vi "Potencia_+_Motor +OSA (1).vi"() -> ()   [LabVIEW 2014]
uses:
  <vilib>/DAQmx/read.llb/DAQmx Read (Analog DBL 1Chan 1Samp).vi
  <vilib>/DAQmx/create/channels.llb/DAQmx Create Channel (AI-Voltage-Basic).vi
  <vilib>/DAQmx/configure/timing.llb/DAQmx Timing (Sample Clock).vi
  <vilib>/Instr/_visa.llb/VISA Configure Serial Port (Instr).vi
  <vilib>/DAQmx/miscellaneous.llb/DAQmx Fill In Error Info.vi
  <vilib>/Utility/file.llb/Write To Spreadsheet File (DBL).vi
panel:
  out "Recibiendo información del OSA":bool
  out "Potencia":dbl[][](array[numeric])
  out "Distancia recorrida":dbl
  out "output array":dbl[][](array[numeric])
  in  "Distancia a recorrer (mm)":dbl=0.5
  in  "Ángulo":string(combo)
  in  "Stop":dbl=1570.0
  in  "Start":dbl=1470.0
  out "Respuesta OSA":string
  out "error out":errorcluster
  out "?":bool
  in  "Atributo":i32(listbox)
  in  "Blank/Disp":bool=TRUE
  in  "Sweep repeat":bool
  in  "Send":bool
  out "Espectro OSA":cluster{dbl[], dbl[]}(graph)
  in  "Trace":i32(listbox)
  in  "Preconfigurar":bool
  in  "Puerto":refnum<visa-resource-name>
  out "Potencia medida":dbl format="%0.2f"
  out "Gráfica de potencia":cluster{dbl[], dbl[]}(graph)
  in  "Índice de refracción":string="Potencia"
  out "size(s)":i32
  in  "Distancia inicial (mm)":dbl=124.65
  out "Tiempo X (S)":dbl
  out "Tiempo Y (S)":dbl format="%#_10g"
  out "Tiempo Z (S)":dbl
  in  "Start/Stop":bool
  in  "COM Config":T1={"VISA resource name"="COM4", "baud rate"=9600, "data bits"=8, "parity"=enum."None", "stop bits"=10, "flow control"=0} {"flow control" items=["None"=0, "XON/XOFF"=1, "RTS/CTS"=2, "DTR/DSR"=4]; "data bits" min=5 max=8 step=1}
  in  "COM Write":string="AA;\nVL0.0000,0.0100,0.0000;\nMR0.0000,-0.5000,0.0000;\nGO;"
  out "Waveform Chart":dbl(graph)
  in  "stop":bool
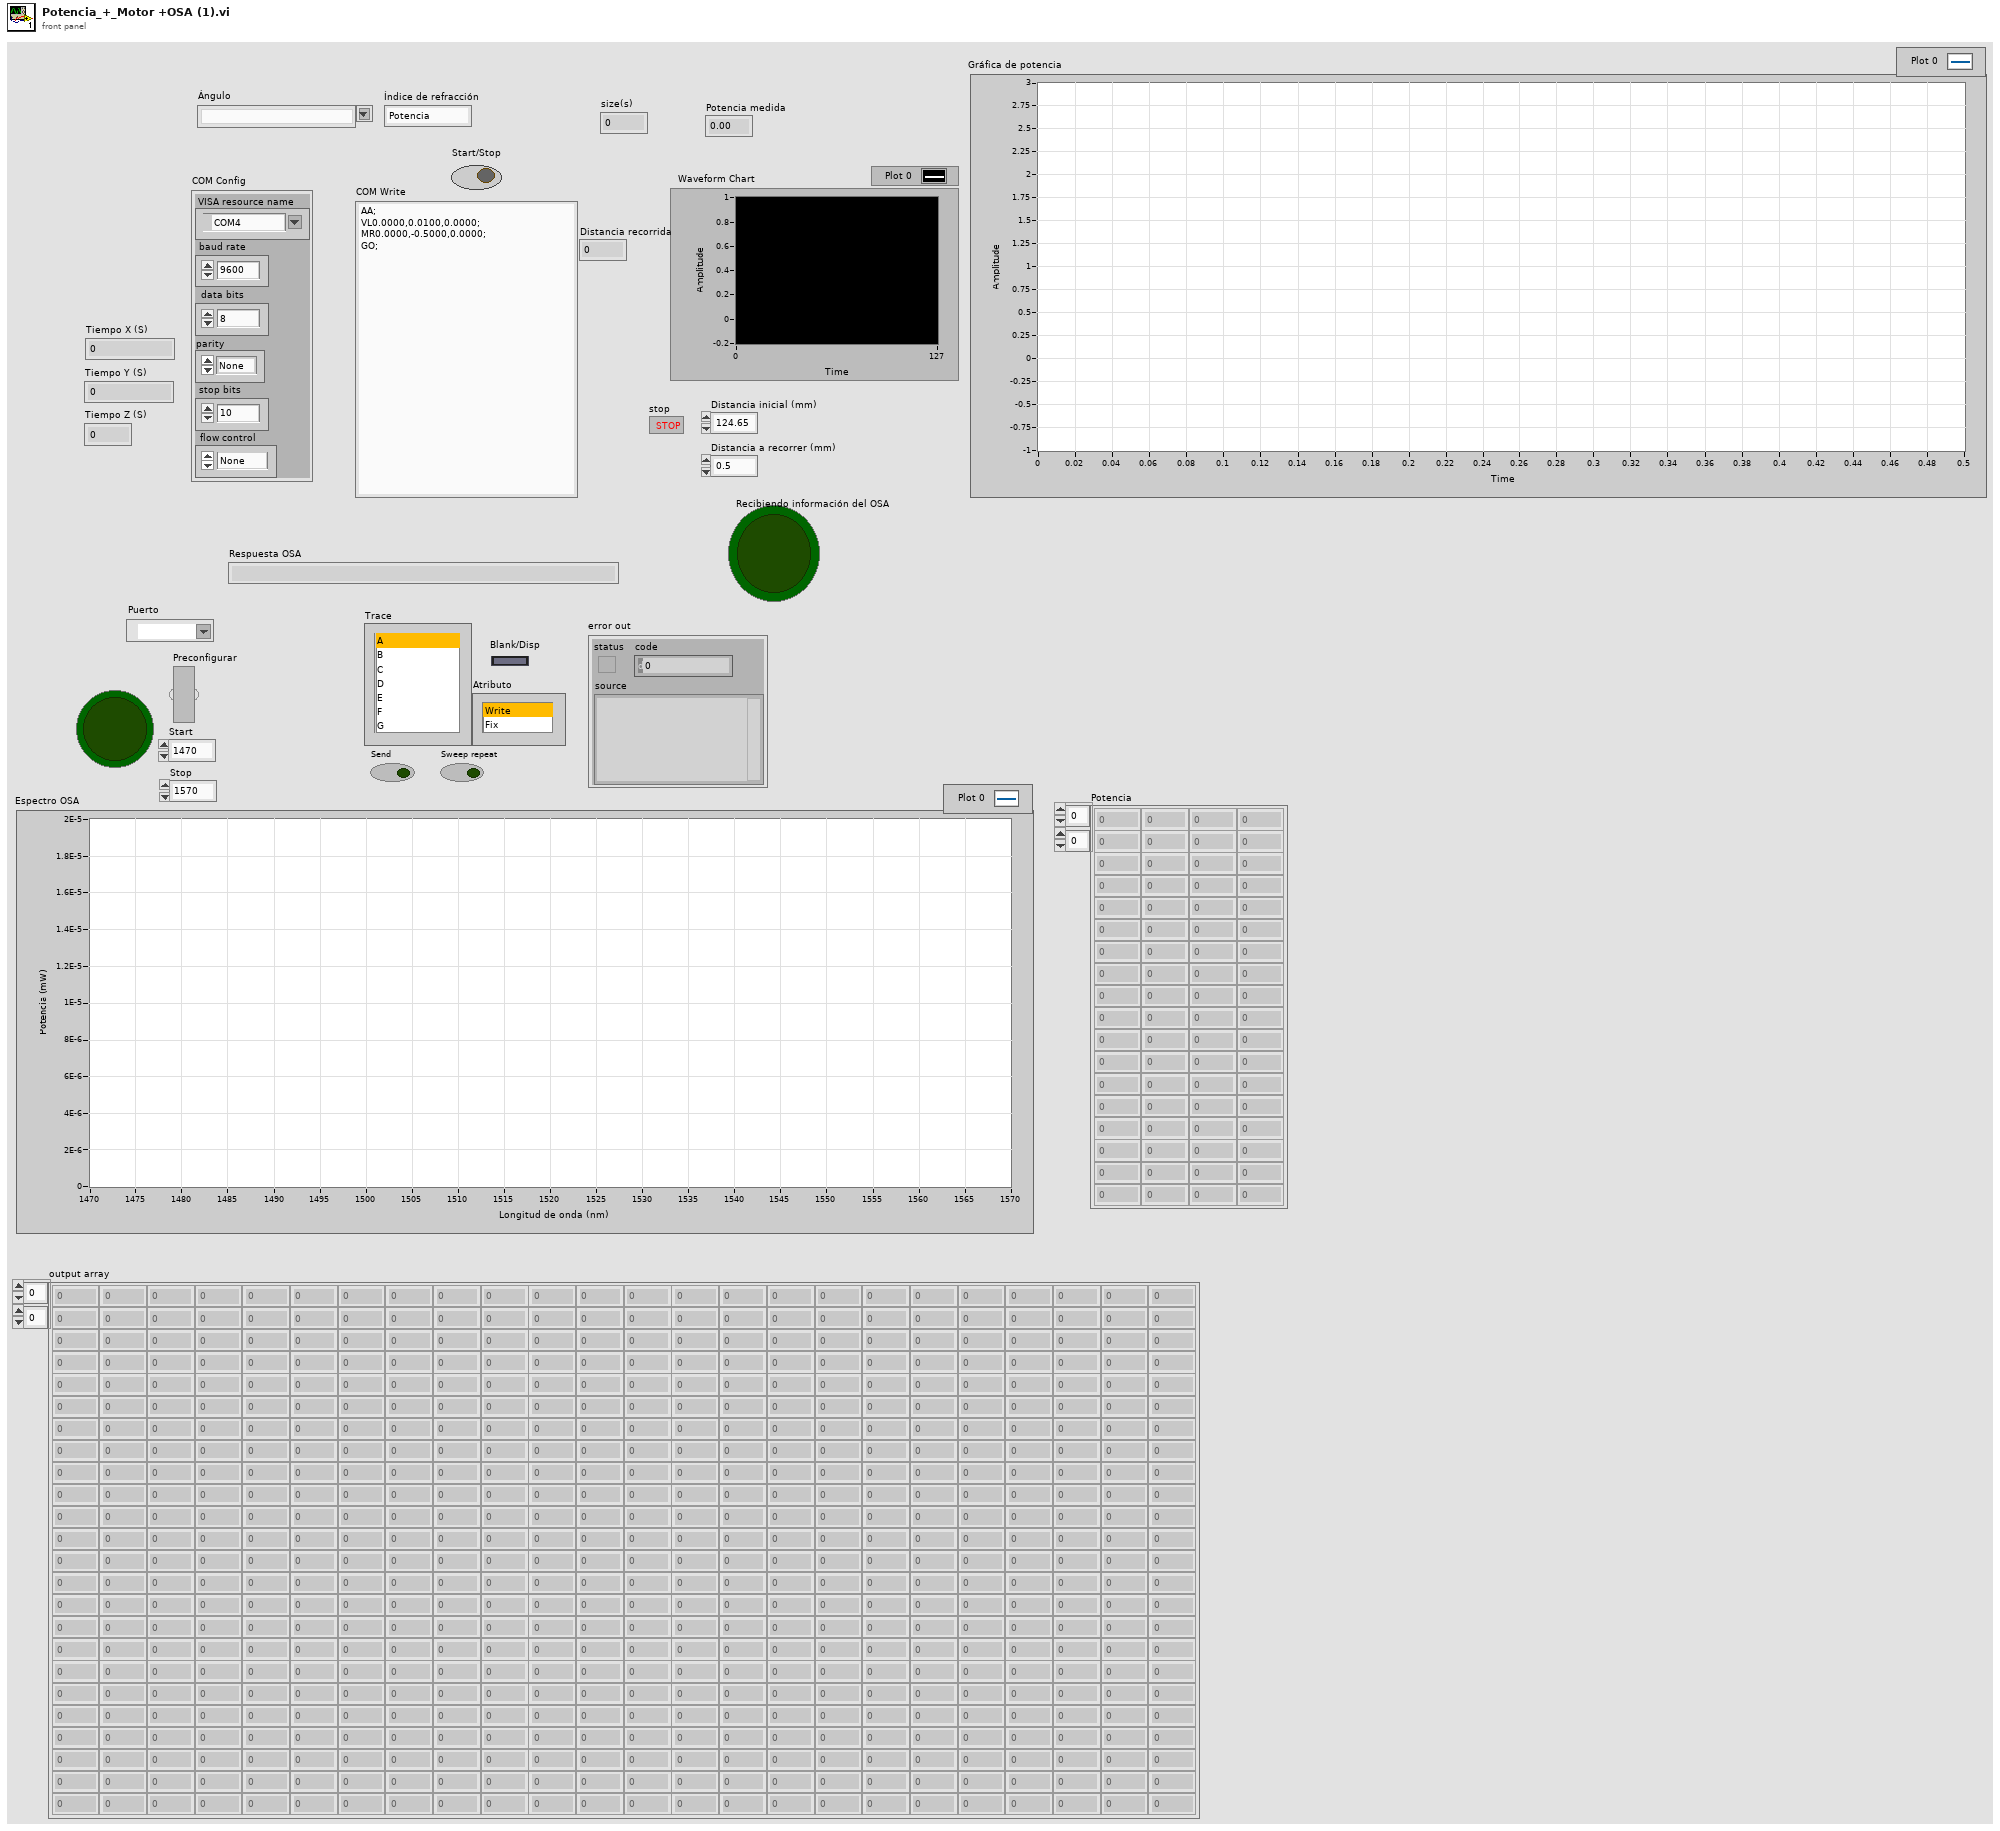
[diagram p1: front panel]
types:
  T1 = cluster{"VISA resource name":refnum<visa-resource-name>, "baud rate":u32, "data bits":u16, "parity":enum16{"None", "Odd", "Even", "Mark", "Space"}, "stop bits":u16, "flow control":u16}
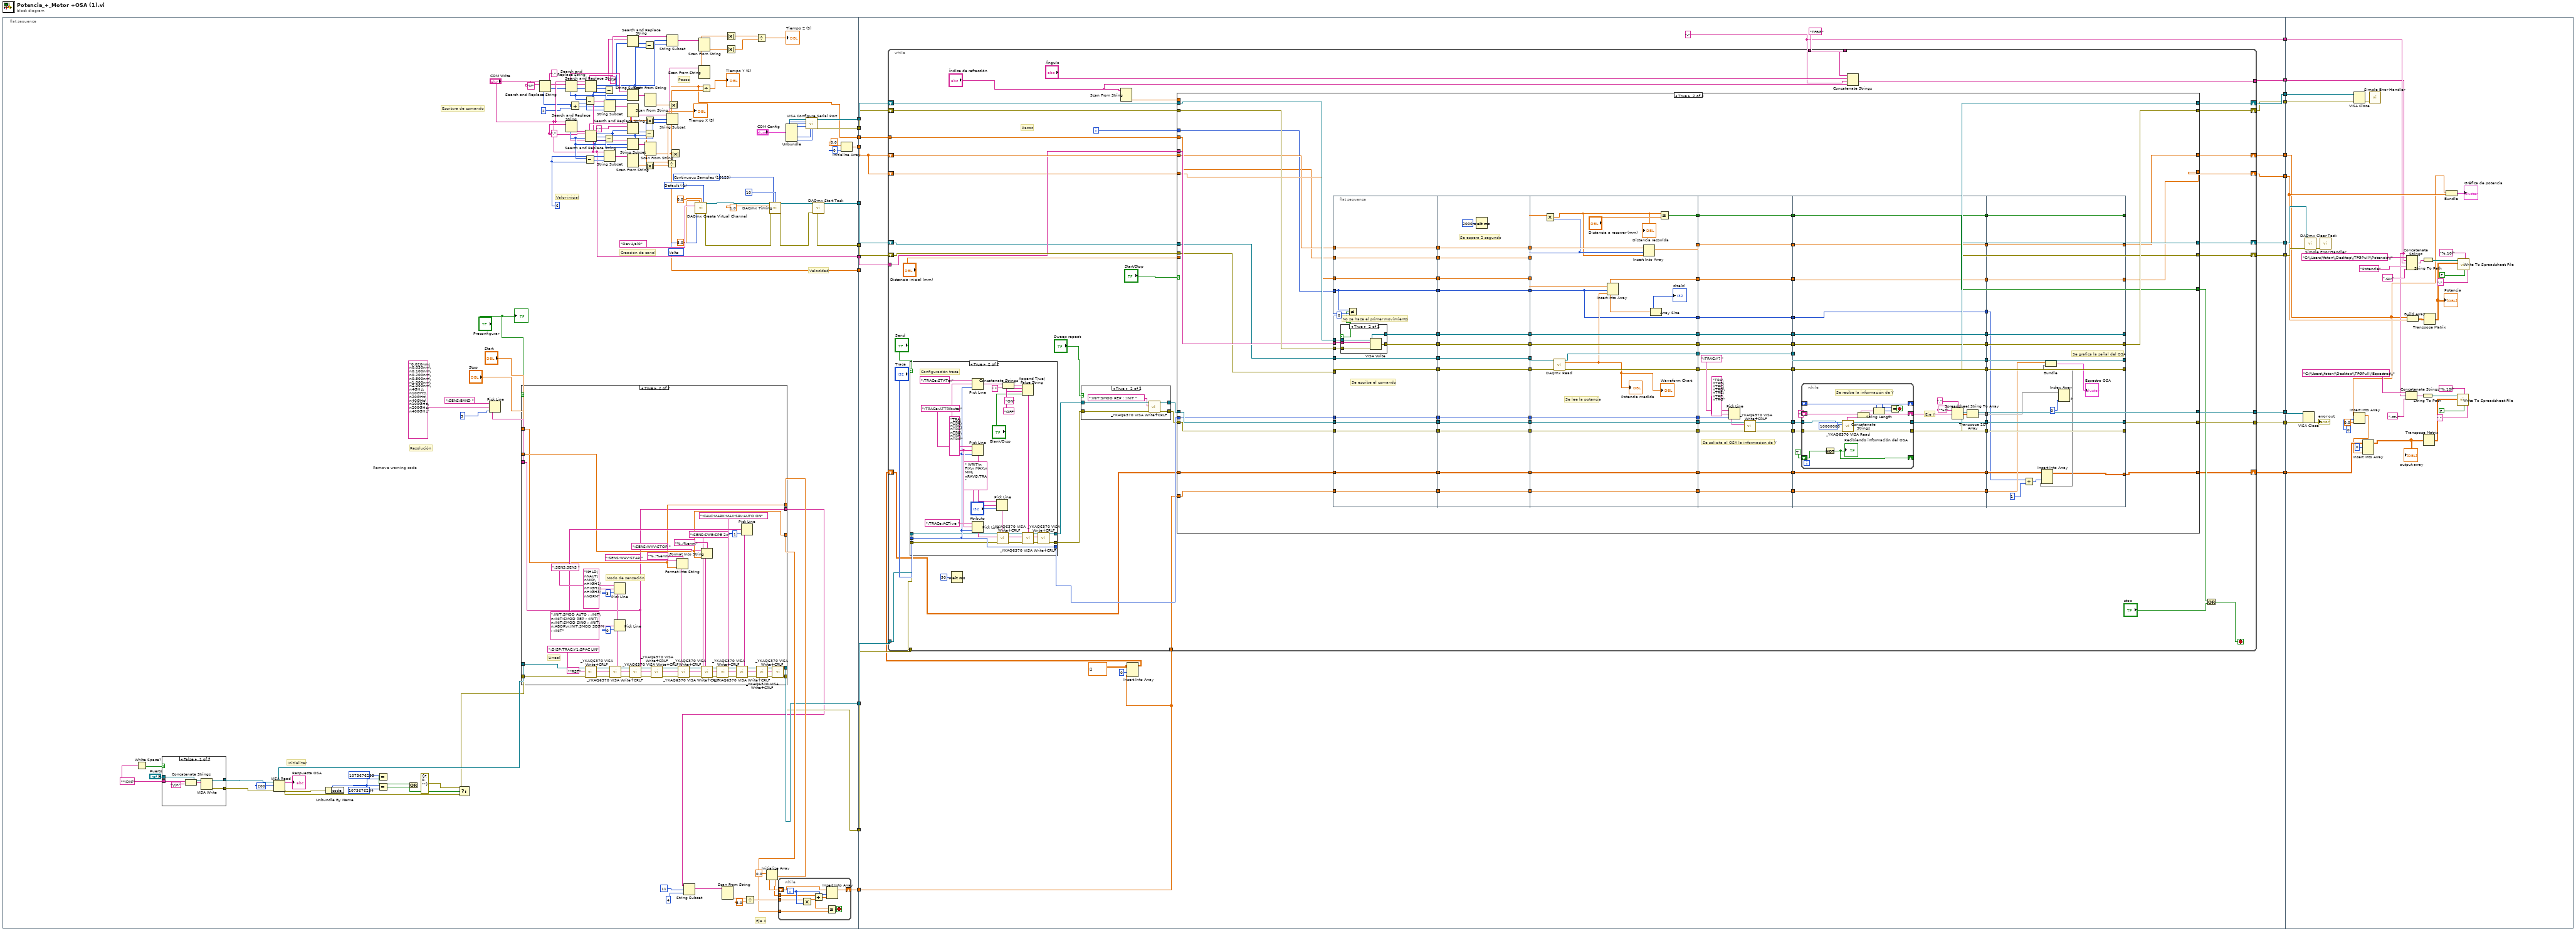
[diagram p0: block diagram]
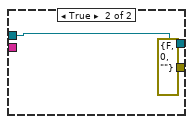
[diagram p3: hidden frame]
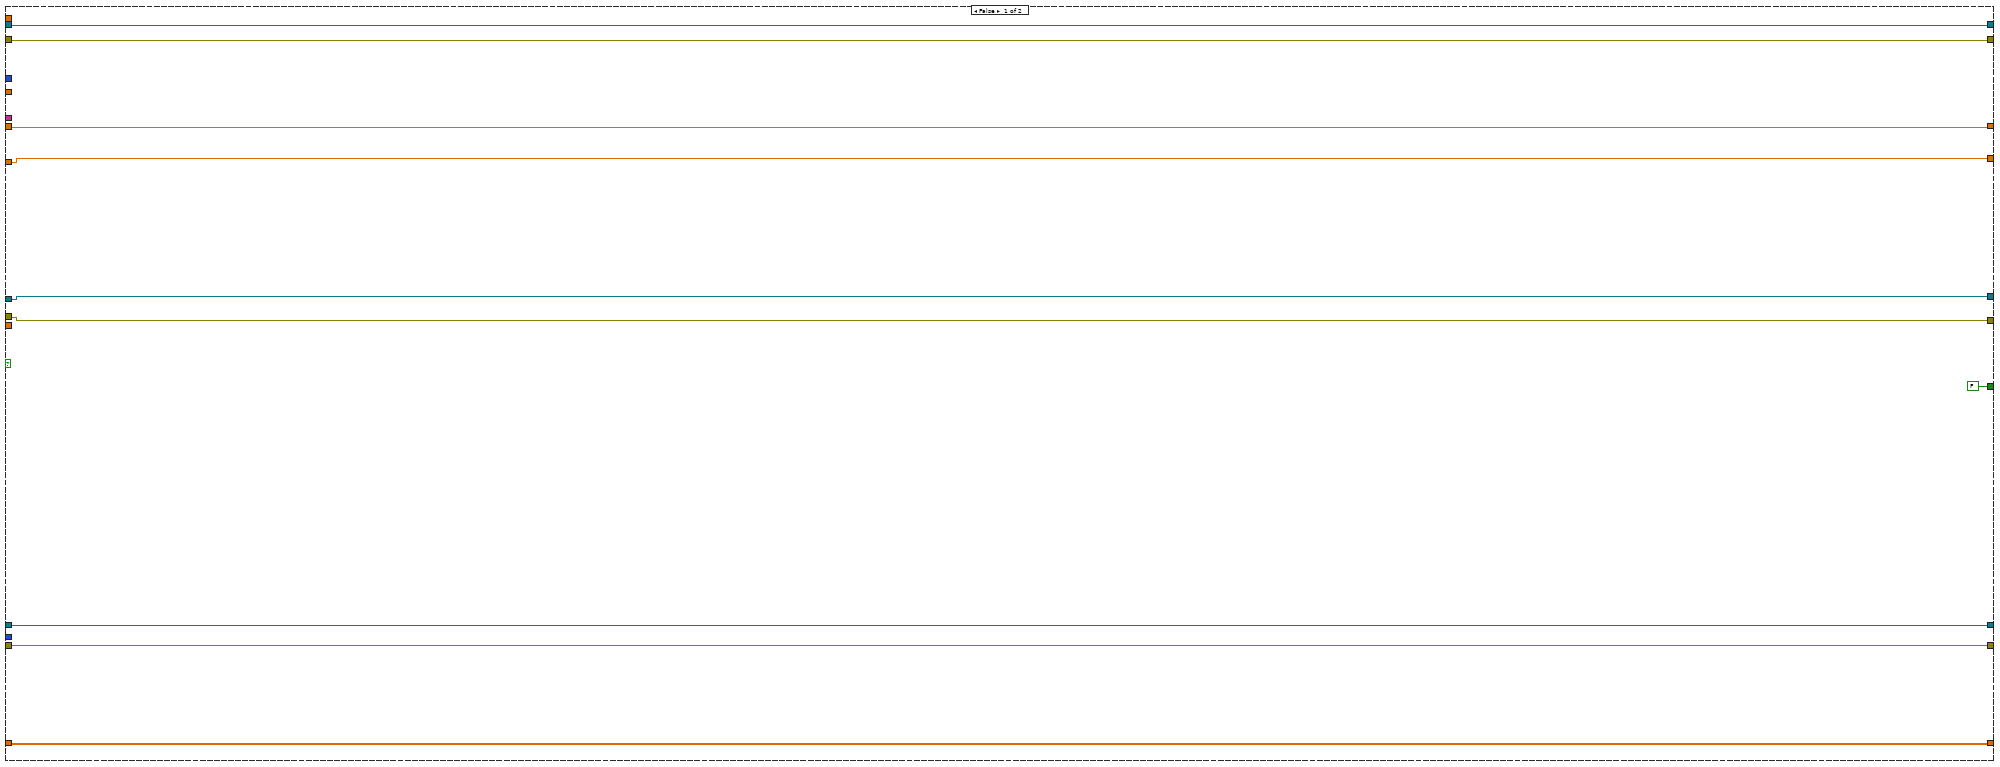
[diagram p6: hidden frame]
diagram:
  n1 = flat-sequence {
    tunnel: [w123] -> w22
    tunnel: [w122] -> w21
    tunnel: [w119] -> w20
    tunnel: [w111] -> w18
    tunnel: [w110] -> w17
    tunnel: ["COM Write"] -> w13
    tunnel: [w28] -> w10
    tunnel: [w27] -> w7
    tunnel: [w26] -> w6
    tunnel: [w25] -> w5
    tunnel: [w24] -> w3
    tunnel: w22 -> [w214]
    tunnel: w21 -> [w226]
    tunnel: w20 -> [w219]
    tunnel: [w218] -> w19
    tunnel: w18 -> [w225]
    tunnel: w17 -> [w224]
    tunnel: [w223] -> w16
    tunnel: [w222] -> w15
    tunnel: [w217] -> w14
    tunnel: w13 -> [w221]
    tunnel: [w216] -> w12
    tunnel: [w215] -> w11
    tunnel: w10 -> [_]
    tunnel: [w213] -> w9
    tunnel: [w212] -> w8
    tunnel: w7 -> [w206]
    tunnel: w6 -> [w211]
    tunnel: w5 -> [w210]
    tunnel: [w209] -> w4
    tunnel: w3 -> [w208]
    tunnel: [w203] -> w2
    tunnel: [w202] -> w1
    tunnel: w19 -> [w553]
    tunnel: w16 -> [w570]
    tunnel: w15 -> [w569]
    tunnel: w14 -> [w537]
    tunnel: w12 -> [w567]
    tunnel: w11 -> [w566]
    tunnel: w9 -> [w564]
    tunnel: w8 -> [w563]
    tunnel: w4 -> [w538]
    tunnel: w2 -> [w544]
    tunnel: w1 -> [w540]
    frame #0 {
      w50 = "*IDN?" ("Strings (empty)")
      w93 = "," ("search string")
      w103 = "," ("search string")
      w109 = 6 ("offset (0)")
      w126 = 10123 items=["Finite Samples"=10178, "Continuous Samples"=10123, "Hardware Timed Single Point"=12522] ("sample mode")
      w131 = -1 items=["Default"=-1, "RSE"=10083, "NRSE"=10078, "Differential"=10106, "Pseudodifferential"=12529] ("input terminal configuration")
      w134 = 10348 items=["Volts"=10348, "From Custom Scale"=10065] ("units")
      # "Pasos"
      # "Eje X"
      # "Resolución"
      # "Inizializar"
      # "Remove warning code"
      # "Velocidad"
      # "Escritura de comando"
      # "Valor inicial"
      # "Creación de canal"
      n2 = White Space?(1:w50) -> (0:w49:bool)
      n3 = case shown="False" w49 {
        tunnel: "Puerto" -> [w197 w201]
        tunnel: [w196 w201] -> w60
        tunnel: w50 -> [w195 _]
        tunnel: [w194 errorcluster {"status"=FALSE, "code"=0, "source"=""} ("error out")] -> w61
        frame False {
          n4 = Concatenate Strings(w195, "\r\n") -> (w198:string)
          n5 = VISA Write(VISA resource name=w197, write buffer=w198) -> (VISA resource name out=w196:refnum<visa-resource-name>, error out=w194:errorcluster)  [unwired: 1 in, 1 out]
        }
        frame True {
        }
      }
      n6 = VISA Read(VISA resource name=w60, byte count=u32 200 ("Byte Count (0)"), error in (no error)=w61) -> (VISA resource name out=w40:refnum<visa-resource-name>, read buffer=→"Respuesta OSA":string, error out=w53:errorcluster)  [unwired: 1 out]
      n7 = Unbundle By Name(w53) -> ("code"=w56:i32)
      n8 = Equal?(x=1073676293, y=w56) -> (x = y?=w57:bool)
      n9 = Equal?(x=1073676294, y=w56) -> (x = y?=w58:bool)
      n10 = Or(x=w57, y=w58) -> (x .or. y?=w59:bool)
      n11 = Select(t=errorcluster {"status"=FALSE, "code"=0, "source"=""}, s=w59, f=w53) -> (s? t:f=w39:errorcluster)
      n12 = Pick Line(string ("")=":SENS:BAND ", multi-line string="0.020nm\n0.050nm\n0.100nm\n0.200nm\n0.500nm\n1.000nm\n2.000nm\n4GHz\n10GHz\n20GHz\n40GHz\n100GHz\n200GHz\n400GHz", line index=3) -> (output string=w47:string)
      n13 = case shown="True" "Preconfigurar" {
        tunnel: w40 -> [w149 w192]
        tunnel: w39 -> [w148 w191]
        tunnel: [w149 w157] -> w26
        tunnel: [w148 w156] -> w25
        tunnel: [w145 w150] -> w23
        tunnel: [w147 w151] -> w30
        tunnel: [w146 w152] -> w29
        tunnel: "Stop" -> [w146 w152]
        tunnel: "Start" -> [w147 w151]
        tunnel: w47 -> [w145 w150]
        frame False {
        }
        frame True {
          w168 = ":INIT:SMOD AUTO ; :INIT\n:INIT:SMOD REP ; :INIT\n:INIT:SMOD SING ; :INIT\n:ABOR\n:INIT:SMOD SEGM ; :INIT"
          # "Lineal"
          # "Modo de sensación"
          n14 = call <instrlib>:"_YKAQ6370 VISA Write+CRLF.vi"("error in (no error)"=w191, "Strings (empty)"="*RST", "VISA resource name"=w192) -> ("error out"=w163:errorcluster, "VISA resource name out"=w164:refnum<visa-resource-name>)  [unwired: 7 in]
          n15 = call <instrlib>:"_YKAQ6370 VISA Write+CRLF.vi"("error in (no error)"=w163, "Strings (empty)"=":DISP:TRAC:Y1:SPAC LIN", "VISA resource name"=w164) -> ("error out"=w160:errorcluster, "VISA resource name out"=w161:refnum<visa-resource-name>)  [unwired: 7 in]
          n16 = Pick Line(string ("")=":SENS:SENS ", multi-line string="NHLD\nNAUT\nMID\nHIGH1\nHIGH2\nHIGH3\nNORM", line index=3) -> (output string=w184:string)
          n17 = Pick Line(multi-line string=w168, line index=0) -> (output string=w172:string)  [unwired: 1 in]
          n18 = call <instrlib>:"_YKAQ6370 VISA Write+CRLF.vi"("error in (no error)"=w160, "Strings (empty)"=w172, "VISA resource name"=w161) -> ("error out"=w173:errorcluster, "VISA resource name out"=w174:refnum<visa-resource-name>)  [unwired: 7 in]
          n19 = call <instrlib>:"_YKAQ6370 VISA Write+CRLF.vi"("error in (no error)"=w173, "Strings (empty)"=w150, "VISA resource name"=w174) -> ("error out"=w188:errorcluster, "VISA resource name out"=w187:refnum<visa-resource-name>)  [unwired: 7 in]
          n20 = Format Into String(format string="%.;%enm", initial string=":SENS:WAV:STAR ", w151) -> (resulting string=w178:string)  [unwired: 1 in, 1 out]
          n21 = call <instrlib>:"_YKAQ6370 VISA Write+CRLF.vi"("error in (no error)"=w188, "Strings (empty)"=w184, "VISA resource name"=w187) -> ("error out"=w189:errorcluster, "VISA resource name out"=w190:refnum<visa-resource-name>)  [unwired: 7 in]
          n22 = Format Into String(format string="%.;%enm", initial string=":SENS:WAV:STOP ", w152) -> (resulting string=w176:string)  [unwired: 1 in, 1 out]
          n23 = call <instrlib>:"_YKAQ6370 VISA Write+CRLF.vi"("error in (no error)"=w189, "Strings (empty)"=w178, "VISA resource name"=w190) -> ("error out"=w181:errorcluster, "VISA resource name out"=w182:refnum<visa-resource-name>)  [unwired: 7 in]
          n24 = call <instrlib>:"_YKAQ6370 VISA Write+CRLF.vi"("error in (no error)"=w181, "Strings (empty)"=w176, "VISA resource name"=w182) -> ("error out"=w158:errorcluster, "VISA resource name out"=w159:refnum<visa-resource-name>)  [unwired: 7 in]
          n25 = call <instrlib>:"_YKAQ6370 VISA Write+CRLF.vi"("error in (no error)"=w158, "Strings (empty)"=":SENS:SWE:SPE 2x", "VISA resource name"=w159) -> ("error out"=w166:errorcluster, "VISA resource name out"=w167:refnum<visa-resource-name>)  [unwired: 7 in]
          n26 = Pick Line(multi-line string=w168, line index=1) -> (output string=w169:string)  [unwired: 1 in]
          n27 = call <instrlib>:"_YKAQ6370 VISA Write+CRLF.vi"("error in (no error)"=w166, "Strings (empty)"=w169, "VISA resource name"=w167) -> ("error out"=w154:errorcluster, "VISA resource name out"=w155:refnum<visa-resource-name>)  [unwired: 7 in]
          n28 = call <instrlib>:"_YKAQ6370 VISA Write+CRLF.vi"("error in (no error)"=w154, "Strings (empty)"=":CALC:MARK:MAX:SRL:AUTO ON", "VISA resource name"=w155) -> ("error out"=w156:errorcluster, "VISA resource name out"=w157:refnum<visa-resource-name>)  [unwired: 7 in]
        }
      }
      n29 = Search and Replace String(input string="COM Write", search string="M" ("replace string (\"\")")) -> (offset past replacement=w84:i32)  [unwired: 6 in, 3 out]
      n30 = Search and Replace String(input string="COM Write", search string=w93, offset=w84) -> (result string=w95:string, offset past replacement=w96:i32)  [unwired: 5 in, 2 out]
      n31 = Search and Replace String(input string="COM Write", search string=w103) -> (result string=w105:string, offset past replacement=w106:i32)  [unwired: 6 in, 2 out]
      n32 = Add(x=w84, y=2) -> (x+y=w82:i32)
      n33 = Subtract(x=w96, y=w82) -> (x-y=w85:i32)
      n34 = Subtract(x=w106, y=w109) -> (x-y=w108:i32)
      n35 = Search and Replace String(input string=w95, search string=w93, offset=w96) -> (result string=w94:string, offset past replacement=w89:i32)  [unwired: 5 in, 2 out]
      n36 = Search and Replace String(input string=w105, search string=w103, offset=w106) -> (result string=w104:string, offset past replacement=w99:i32)  [unwired: 5 in, 2 out]
      n37 = Subtract(x=w89, y=w96) -> (x-y=w97:i32)
      n38 = Subtract(x=w99, y=w106) -> (x-y=w107:i32)
      n39 = String Subset(string="COM Write", offset (0)=w82, length (rest)=w85) -> (substring=w64:string)
      n40 = String Subset(string="COM Write", offset (0)=w109, length (rest)=w108) -> (substring=w63:string)
      n41 = Search and Replace String(input string=w94, search string=";", offset=w89) -> (result string=w92:string, offset past replacement=w90:i32)  [unwired: 5 in, 2 out]
      n42 = String Subset(string=w95, offset (0)=w96, length (rest)=w97) -> (substring=w68:string)
      n43 = Scan From String(input string=w64) -> (output 1=w76:dbl)  [unwired: 4 in, 3 out]
      n44 = Search and Replace String(input string=w104, search string=";", offset=w99) -> (result string=w102:string, offset past replacement=w100:i32)  [unwired: 5 in, 2 out]
      n45 = String Subset(string=w105, offset (0)=w106, length (rest)=w107) -> (substring=w67:string)
      n46 = Scan From String(input string=w63) -> (output 1=w79:dbl)  [unwired: 4 in, 3 out]
      n47 = Subtract(x=w90, y=w89) -> (x-y=w91:i32)
      n48 = Subtract(x=w100, y=w99) -> (x-y=w101:i32)
      n49 = Absolute Value(x=w76) -> (abs(x)=w77:dbl)
      n50 = Absolute Value(x=w79) -> (abs(x)=w78:dbl)
      n51 = Scan From String(input string=w68) -> (output 1=w71:dbl)  [unwired: 4 in, 3 out]
      n52 = Scan From String(input string=w67) -> (output 1=w70:dbl)  [unwired: 4 in, 3 out]
      n53 = Divide(x=w77, y=w78) -> (x/y=→"Tiempo X (S)":dbl)
      n54 = String Subset(string=w92, offset (0)=w89, length (rest)=w91) -> (substring=w66:string)
      n55 = String Subset(string=w102, offset (0)=w99, length (rest)=w101) -> (substring=w65:string)
      n56 = Absolute Value(x=w71) -> (abs(x)=w24:dbl)
      n57 = Absolute Value(x=w70) -> (abs(x)=w28:dbl)
      n58 = String Subset(string=w23, offset (0)=11, length (rest)=4 ("length (rest)")) -> (substring=w37:string)
      n59 = call-poly <vilib>:"DAQmx Create Virtual Channel.vi"("maximum value"=5.0, "minimum value"=0.0, "input terminal configuration"=w131, "physical channels"=tag "Dev4/ai0", "units"=w134) -> ("task out"=w130:refnum<k21>, "error out"=w129:errorcluster)  [unwired: 9 in]
      n60 = Scan From String(input string=w66) -> (output 1=w75:dbl)  [unwired: 4 in, 3 out]
      n61 = Scan From String(input string=w65) -> (output 1=w73:dbl)  [unwired: 4 in, 3 out]
      n62 = Divide(x=w24, y=w28) -> (x/y=→"Tiempo Y (S)":dbl)
      n63 = Scan From String(input string=w37) -> (output 1=w33:dbl)  [unwired: 4 in, 3 out]
      n64 = Absolute Value(x=w75) -> (abs(x)=w74:dbl)
      n65 = Absolute Value(x=w73) -> (abs(x)=w72:dbl)
      n66 = Divide(x=w33, y=5.0) -> (x/y=w32:dbl)
      n67 = Divide(x=w74, y=w72) -> (x/y=→"Tiempo Z (S)":dbl)
      n68 = Initialize Array(0.0 ("element")) -> (w36:dbl[])  [unwired: 1 in]
      n69 = call-poly <vilib>:"DAQmx Timing.vi"("task/channels in"=w130, "sample mode"=w126, "samples per channel"=10, "rate"=1.0, "error in"=w129) -> ("task out"=w125:refnum<k21>, "error out"=w124:errorcluster)  [unwired: 9 in]
      n70 = while {
        shift-right: [w143] -> w27
        shift-left: w36 -> [w144]
        tunnel: w30 -> [w139]
        tunnel: w32 -> [w141]
        tunnel: w29 -> [w137]
        i -> [w142]
        stop <- w136 stop-if-true
        n71 = Multiply(x=w141, y=w142) -> (x*y=w140:dbl)
        n72 = Add(x=w139, y=w140) -> (x+y=w138:dbl)
        n73 = Greater Or Equal?(x=w138, y=w137) -> (x >= y?=w136:bool)
        n74 = Insert Into Array(array=w144, index=w142, new element=w138) -> (w143:dbl[])
      }
      n75 = Unbundle("COM Config") -> ("VISA resource name"=w113:refnum<visa-resource-name>, "baud rate"=w114:u32, "data bits"=w115:u16, "parity"=w118:enum16{"None", "Odd", "Even", "Mark", "Space"}, "stop bits"=w116:u16, "flow control"=w117:u16)
      n76 = call-poly "VISA Configure Serial Port"("VISA resource name"=w113, "baud rate (9600)"=w114, "data bits (8)"=w115, "parity (0:none)"=w118, "stop bits (10: 1 bit)"=w116, "flow control (0:none)"=w117) -> ("VISA resource name out"=w111:refnum<visa-resource-name>, "error out"=w110:errorcluster)  [unwired: 8 in]
      n77 = call <vilib>:"DAQmx Start Task.vi"("task/channels in"=w125, "error in"=w124) -> ("task out"=w123:refnum<k21>, "error out"=w122:errorcluster)  [unwired: 12 in]
      n78 = Initialize Array(0.0 ("element"), 0 ("dimension size")) -> (w119:dbl[])
      "?" <- "Preconfigurar"
    }
    frame #1 {
      w202 = "-"
      n79 = Insert Into Array(array=dbl[][] [], index (col)=0 ("disabled index (col)"), new element=w206) -> (w204:dbl[][])  [unwired: 1 in]
      n80 = while {
        shift-right: [w253] -> w217
        shift-left: w219 -> [w268]
        shift-right: [w265] -> w223
        shift-left: w225 -> [w262]
        shift-right: [w264] -> w222
        shift-left: w224 -> [w266]
        tunnel: w221 -> [w261]
        tunnel: [w256] -> w209
        tunnel: "TFBG" -> [w259]
        tunnel: w202 -> [w257]
        shift-right: [w254] -> w218
        shift-left: w219 -> [w255]
        shift-right: [w252] -> w216
        shift-left: w214 -> [w250]
        shift-right: [w251] -> w215
        shift-left: w226 -> [w267]
        tunnel: [w242] -> w213
        tunnel: [w241] -> w212
        tunnel: w211 -> [w240]
        tunnel: w210 -> [w239]
        tunnel: w208 -> [w237]
        tunnel: w206 -> [w231]
        shift-right: [w230] -> w203
        shift-left: w204 -> [w229]
        i -> [w236]
        stop <- w233 stop-if-true
        # "Pasos"
        n81 = case shown="True" "Send" {
          tunnel: [w277 w284] -> w238
          tunnel: [w276 w283] -> w248
          tunnel: [w278 w281] -> w243
          tunnel: "Trace" -> [w278 w281]
          tunnel: w240 -> [w277 w280]
          tunnel: w239 -> [w276 w279]
          frame False {
          }
          frame True {
            w286 = "TRA\nTRB\nTRC\nTRD\nTRE\nTRF\nTRG"
            # "Configuración trace"
            n82 = Pick Line(string ("")=":TRACe:STATe:", multi-line string=w286, line index=w281) -> (output string=w287:string)
            n83 = Pick Line(string ("")=":TRACe:ATTRibute:", multi-line string=w286, line index=w281) -> (output string=w292:string)
            n84 = Pick Line(string ("")=":TRACe:ACTive ", multi-line string=w286, line index=w281) -> (output string=w288:string)
            n85 = Pick Line(string ("")=w292, multi-line string=" WRIT\n FIX\n MAX\n MIN\nRAVG:TRA ", line index="Atributo") -> (output string=w291:string)
            n86 = call <instrlib>:"_YKAQ6370 VISA Write+CRLF.vi"("error in (no error)"=w279, "Strings (empty)"=w288, "VISA resource name"=w280) -> ("error out"=w300:errorcluster, "VISA resource name out"=w299:refnum<visa-resource-name>)  [unwired: 7 in]
            n87 = Concatenate Strings(w287, " " ("string")) -> (w290:string)
            n88 = Append True/False String(1:"Blank/Disp", 2:"OFF", 3:"ON", 4:w290) -> (0:w296:string)
            n89 = call <instrlib>:"_YKAQ6370 VISA Write+CRLF.vi"("error in (no error)"=w300, "Strings (empty)"=w291, "VISA resource name"=w299) -> ("error out"=w297:errorcluster, "VISA resource name out"=w298:refnum<visa-resource-name>)  [unwired: 7 in]
            n90 = call <instrlib>:"_YKAQ6370 VISA Write+CRLF.vi"("error in (no error)"=w297, "Strings (empty)"=w296, "VISA resource name"=w298) -> ("error out"=w283:errorcluster, "VISA resource name out"=w284:refnum<visa-resource-name>)  [unwired: 7 in]
          }
        }
        n91 = Wait (ms)(milliseconds to wait=u32 50) -> ()  [unwired: 1 out]
        n92 = case shown="True" "Sweep repeat" {
          tunnel: w238 -> [w270 w275]
          tunnel: w248 -> [w269 w274]
          tunnel: [w270 w272] -> w244
          tunnel: [w269 w271] -> w232
          frame False {
          }
          frame True {
            n93 = call <instrlib>:"_YKAQ6370 VISA Write+CRLF.vi"("error in (no error)"=w274, "Strings (empty)"=":INIT:SMOD REP ; :INIT ", "VISA resource name"=w275) -> ("error out"=w271:errorcluster, "VISA resource name out"=w272:refnum<visa-resource-name>)  [unwired: 7 in]
          }
        }
        n94 = Scan From String(input string="Índice de refracción") -> (output 1=w228:dbl)  [unwired: 4 in, 3 out]
        n95 = case shown="True" "Start/Stop" {
          tunnel: w250 -> [w311 w382]
          tunnel: w268 -> [w308 w367]
          tunnel: w267 -> [w310 w381]
          tunnel: [w309 w371] -> w254
          tunnel: w262 -> [w313 w391]
          tunnel: w266 -> [w312 w390]
          tunnel: [w313 w384] -> w265
          tunnel: [w312 w383] -> w264
          tunnel: [w308 w368] -> w253
          tunnel: w261 -> [_ w389]
          tunnel: "Distancia inicial (mm)" -> [_ _]
          tunnel: w255 -> [w309 w374]
          tunnel: [w311 w376] -> w252
          tunnel: [w310 w375] -> w251
          tunnel: w244 -> [w307 w399]
          tunnel: w232 -> [w306 w398]
          tunnel: w243 -> [_ w397]
          tunnel: [w307 w396] -> w242
          tunnel: [w306 w395] -> w241
          tunnel: w237 -> [_ w365]
          tunnel: w236 -> [_ w366]
          tunnel: [FALSE w362] -> w234
          tunnel: w229 -> [w304 w329]
          tunnel: w231 -> [_ w328]
          tunnel: [w304 w314] -> w230
          tunnel: w228 -> [_ _]
          frame False {
          }
          frame True {
            n96 = flat-sequence {
              tunnel: w397 -> [w417]
              tunnel: w398 -> [w418]
              tunnel: w399 -> [w419]
              tunnel: [w419] -> w361
              tunnel: [w418] -> w359
              tunnel: [w417] -> w357
              tunnel: w391 -> [w416]
              tunnel: w390 -> [w415]
              tunnel: w389 -> [w414]
              tunnel: [w413] -> w355
              tunnel: [w412] -> w353
              tunnel: w382 -> [w411]
              tunnel: [w411] -> w351
              tunnel: w381 -> [w410]
              tunnel: [w410] -> w349
              tunnel: w374 -> [w409]
              tunnel: [w409] -> w347
              tunnel: w367 -> [w408]
              tunnel: [w408] -> w345
              tunnel: w366 -> [w406]
              tunnel: [w406] -> w343
              tunnel: w365 -> [w407]
              tunnel: [w407] -> w341
              tunnel: w329 -> [w402]
              tunnel: w328 -> [w403]
              tunnel: [w403] -> w323
              tunnel: [w402] -> w318
              tunnel: w361 -> [w440]
              tunnel: [w440] -> w360
              tunnel: w359 -> [w439]
              tunnel: [w439] -> w358
              tunnel: w357 -> [w438]
              tunnel: [w438] -> w356
              tunnel: w355 -> [w437]
              tunnel: [w437] -> w354
              tunnel: w353 -> [w436]
              tunnel: [w436] -> w352
              tunnel: w351 -> [w435]
              tunnel: [w435] -> w350
              tunnel: w349 -> [w434]
              tunnel: [w434] -> w348
              tunnel: w347 -> [w433]
              tunnel: [w433] -> w346
              tunnel: w345 -> [w432]
              tunnel: [w432] -> w344
              tunnel: w343 -> [w431]
              tunnel: [w431] -> w342
              tunnel: w341 -> [w430]
              tunnel: [w430] -> w340
              tunnel: [w428] -> w324
              tunnel: w323 -> [w428]
              tunnel: [w427] -> w319
              tunnel: w318 -> [w427]
              tunnel: [w462] -> w394
              tunnel: [w461] -> w393
              tunnel: [w460] -> w392
              tunnel: w360 -> [w462]
              tunnel: w358 -> [w461]
              tunnel: w356 -> [w460]
              tunnel: [w459] -> w387
              tunnel: w354 -> [w459]
              tunnel: [w458] -> w385
              tunnel: w352 -> [w458]
              tunnel: w350 -> [w457]
              tunnel: w348 -> [w456]
              tunnel: [w455] -> w379
              tunnel: [w454] -> w377
              tunnel: w346 -> [w453]
              tunnel: [w451] -> w372
              tunnel: w344 -> [w449]
              tunnel: [w448] -> w369
              tunnel: w342 -> [w442]
              tunnel: w340 -> [w446]
              tunnel: [w445] -> w363
              tunnel: [w444] -> w325
              tunnel: w324 -> [w444]
              tunnel: [w443] -> w320
              tunnel: w319 -> [w443]
              tunnel: [w442] -> w315
              tunnel: [w478] -> w401
              tunnel: [w477] -> w400
              tunnel: w394 -> [w480]
              tunnel: w393 -> [w479]
              tunnel: w392 -> [w473]
              tunnel: [w472] -> w388
              tunnel: w387 -> [w472]
              tunnel: [w471] -> w386
              tunnel: w385 -> [w471]
              tunnel: [w470] -> w380
              tunnel: w379 -> [w470]
              tunnel: [w469] -> w378
              tunnel: w377 -> [w469]
              tunnel: [w468] -> w373
              tunnel: w372 -> [w468]
              tunnel: [w467] -> w370
              tunnel: w369 -> [w467]
              tunnel: [w466] -> w364
              tunnel: w363 -> [w466]
              tunnel: [w465] -> w326
              tunnel: w325 -> [w465]
              tunnel: [w464] -> w321
              tunnel: w320 -> [w464]
              tunnel: [w463] -> w316
              tunnel: w315 -> [w463]
              tunnel: w401 -> [w501]
              tunnel: w400 -> [w500]
              tunnel: w388 -> [w491]
              tunnel: w386 -> [w490]
              tunnel: w380 -> [w489]
              tunnel: w378 -> [w488]
              tunnel: w373 -> [w487]
              tunnel: w370 -> [w486]
              tunnel: w364 -> [w485]
              tunnel: [w494] -> w339
              tunnel: [w493] -> w338
              tunnel: [w492] -> w337
              tunnel: [w491] -> w336
              tunnel: [w490] -> w335
              tunnel: [w489] -> w334
              tunnel: [w488] -> w333
              tunnel: [w487] -> w332
              tunnel: [w486] -> w331
              tunnel: [w485] -> w330
              tunnel: [w484] -> w327
              tunnel: w326 -> [w484]
              tunnel: [w483] -> w322
              tunnel: w321 -> [w483]
              tunnel: [w482] -> w317
              tunnel: w316 -> [w482]
              tunnel: [w525] -> w362
              tunnel: [w526] -> w368
              tunnel: [w527] -> w371
              tunnel: [w528] -> w375
              tunnel: [w529] -> w376
              tunnel: [w530] -> w383
              tunnel: [w531] -> w384
              tunnel: [w532] -> w395
              tunnel: [w533] -> w396
              tunnel: w339 -> [w524]
              tunnel: w338 -> [w533]
              tunnel: w337 -> [w532]
              tunnel: w336 -> [w531]
              tunnel: w335 -> [w530]
              tunnel: w334 -> [w529]
              tunnel: w333 -> [w528]
              tunnel: w332 -> [w527]
              tunnel: w331 -> [w526]
              tunnel: w330 -> [w525]
              tunnel: w327 -> [w522]
              tunnel: w322 -> [w520]
              tunnel: w317 -> [w518]
              tunnel: [w516] -> w314
              frame #0 {
                # "No se hace el primer movimiento"
                # "Se escribe el comando"
                n97 = Not Equal?(x=w406, y=0) -> (x != y?=w404:bool)
                n98 = case shown="True" w404 {
                  tunnel: w416 -> [w421 w426]
                  tunnel: w415 -> [w420 w425]
                  tunnel: w414 -> [_ w424]
                  tunnel: [w421 w423] -> w413
                  tunnel: [w420 w422] -> w412
                  frame False {
                  }
                  frame True {
                    n99 = VISA Write(VISA resource name=w426, write buffer=w424, error in (no error)=w425) -> (VISA resource name out=w423:refnum<visa-resource-name>, error out=w422:errorcluster)  [unwired: 1 out]
                  }
                }
              }
              frame #1 {
                # "Se espera 2 segundo"
                n100 = Wait (ms)(milliseconds to wait=u32 2000) -> ()  [unwired: 1 out]
              }
              frame #2 {
                # "Se lee la potencia"
                n101 = Multiply(x=w446, y=w442) -> (x*y=w441:dbl)
                "Distancia recorrida" <- w441
                n102 = call-poly <vilib>:"DAQmx Read.vi"("task/channels in"=w457, "error in"=w456) -> ("task out"=w455:refnum<k21>, "data"=w450:dbl, "error out"=w454:errorcluster)  [unwired: 11 in]
                "Potencia medida" <- w450
                "Waveform Chart" <- w450
                n103 = Insert Into Array(array=w453, index=w442, new element=w450) -> (w451:dbl[])
                n104 = Insert Into Array(array=w449, index=w442, new element=w441) -> (w448:dbl[])
                n105 = Array Size(array=w451) -> (size(s)=→"size(s)":i32)
                n106 = Greater Or Equal?(x=w441, y="Distancia a recorrer (mm)") -> (x >= y?=w445:bool)
              }
              frame #3 {
                # "Se solicita al OSA la información de Y"
                n107 = Pick Line(string ("")=":TRAC:Y? " ("Strings (empty)"), multi-line string="TRA\nTRB\nTRC\nTRD\nTRE\nTRF\nTRG", line index=w473) -> (output string=w474:string)
                n108 = call <instrlib>:"_YKAQ6370 VISA Write+CRLF.vi"("error in (no error)"=w479, "Strings (empty)"=w474, "VISA resource name"=w480) -> ("error out"=w477:errorcluster, "VISA resource name out"=w478:refnum<visa-resource-name>)  [unwired: 7 in]
              }
              frame #4 {
                # "Eje Y"
                n109 = while {
                  tunnel: w501 -> [w513]
                  tunnel: w500 -> [w512]
                  tunnel: [w511] -> w493
                  tunnel: [w510] -> w492
                  shift-right: [w504] -> w498
                  shift-left: "" -> [w509]
                  shift-right: [w506] -> _
                  shift-left: _ -> [w507]
                  shift-right: [w502] -> _
                  shift-left: TRUE -> [w503]
                  stop <- w505 stop-if-true
                  # "Se recibe la información de Y"
                  n110 = Not(x=w503) -> (.not. x?=w502:bool)
                  "Recibiendo información del OSA" <- w502
                  n111 = call <instrlib>:"_YKAQ6370 VISA Read.vi"("error in (no error)"=w512, "Byte Count (0)"=u32 10000000, "VISA resource name"=w513) -> ("error out"=w510:errorcluster, "Read Data"=w508:string, "VISA resource name out"=w511:refnum<visa-resource-name>)  [unwired: 5 in, 1 out]
                  n112 = Concatenate Strings(w509, w508) -> (w504:string)
                  n113 = String Length(string=w504) -> (length=w506:i32)
                  n114 = Equal?(x=w507, y=w506) -> (x = y?=w505:bool)
                }
                n115 = Spreadsheet String To Array(delimiter (Tab)=",", format string="%s", spreadsheet string=w498) -> (array=w495:dbl[][])  [unwired: 1 in]
                n116 = Transpose 2D Array(2D array=w495) -> (transposed array=w494:dbl[][])
              }
              frame #5 {
                # "Se grafica la señal del OSA"
                n117 = Add(x=w518, y=1) -> (x+y=w515:i32)
                n118 = Index Array(array=w524, index (col)=0 ("disabled index (col)")) -> (element=w519:dbl[])  [unwired: 1 in]
                n119 = Insert Into Array(array=w520, index (col)=w515, new element=w519) -> (w516:dbl[][])  [unwired: 1 in]
                n120 = Bundle(w522, w519) -> (→"Espectro OSA":cluster{dbl[], dbl[]})  [unwired: 1 in]
              }
            }
          }
        }
        n121 = Concatenate Strings(w259, "Ángulo", w257, "Índice de refracción") -> (w256:string)
        n122 = Or(x=w234, y="stop") -> (x .or. y?=w233:bool)
      }
    }
    frame #2 {
      n123 = VISA Close(VISA resource name=w564, error in (no error)=w563) -> (error out=→"error out":errorcluster)
      n124 = call <vilib>:"DAQmx Clear Task.vi"("task in"=w567, "error in"=w566) -> ("error out"=w568:errorcluster)  [unwired: 13 in]
      n125 = call <vilib>:"Simple Error Handler.vi"("error in (no error)"=w568) -> ()  [unwired: 4 in, 5 out]
      n126 = VISA Close(VISA resource name=w570, error in (no error)=w569) -> (error out=w571:errorcluster)
      n127 = Insert Into Array(array=w537, index=0, new element=0.0 ("new element/subarray")) -> (w536:dbl[])
      n128 = Insert Into Array(array=w544, index (row)=0, new element=w536) -> (w542:dbl[][])  [unwired: 1 in]
      "output array" <- w542
      n129 = call <vilib>:"Simple Error Handler.vi"("error in (no error)"=w571) -> ()  [unwired: 4 in, 5 out]
      n130 = Concatenate Strings("C:\\Users\\foton\\Desktop\\TFGPull\\Espectros\\" ("string"), w538, ".csv" ("string")) -> (w549:string)
      n131 = Concatenate Strings("C:\\Users\\foton\\Desktop\\TFGPull\\Potencia\\" ("string"), w538, w540, "Potencia" ("string"), ".csv" ("string")) -> (w558:string)
      n132 = Build Array(w537, w553) -> (w561:dbl[][])
      n133 = String To Path(string=w549) -> (path=w550:path)
      n134 = String To Path(string=w558) -> (path=w559:path)
      n135 = Transpose Matrix(1:w542) -> (0:w552:dbl[][])
      n136 = Transpose Matrix(1:w561) -> (0:w560:dbl[][])
      "Potencia" <- w560
      n137 = Bundle(w537, w553) -> (→"Gráfica de potencia":cluster{dbl[], dbl[]})  [unwired: 1 in]
      n138 = call-poly <vilib>:"Write To Spreadsheet File.vi"("delimiter (\\t)"="," ("delimiter (\\t)"), "transpose? (no:F)"=FALSE, "format (%.3f)"="%.10f", "2D data"=w552, "file path (dialog if empty)"=w550) -> ()  [unwired: 3 in, 1 out]
      n139 = call-poly <vilib>:"Write To Spreadsheet File.vi"("delimiter (\\t)"="," ("delimiter (\\t)"), "transpose? (no:F)"=FALSE, "format (%.3f)"="%.10f", "2D data"=w560, "file path (dialog if empty)"=w559) -> ()  [unwired: 3 in, 1 out]
    }
  }
